vi "EminemGlobals.vi"() -> ()   [LabVIEW 2023]
uses:
  EminemStatesEnum.ctl
panel:
  out "ShooterSpeedRPM_FB":dbl=4000.0
  out "RShooterMotorOutput":dbl
  out "LShooterMotorOutput":dbl
  out "RShooterFilteredSpeed":dbl
  out "RShooterSpeed":dbl
  out "LShooterFilteredSpeed":dbl
  out "LShooterSpeed":dbl
  out "M&M_State":T1=enum."13-AmpDone"
  out "RAtSpeed":bool
  out "LAtSpeed":bool
  out "ShooterSensor":bool
  out "IntakeSensor":bool
  out "IntakeGetNoteMotorDMD":dbl=0.5
  out "ShooterSpeedRPM":dbl=4000.0
  out "ReadyForCommand":bool
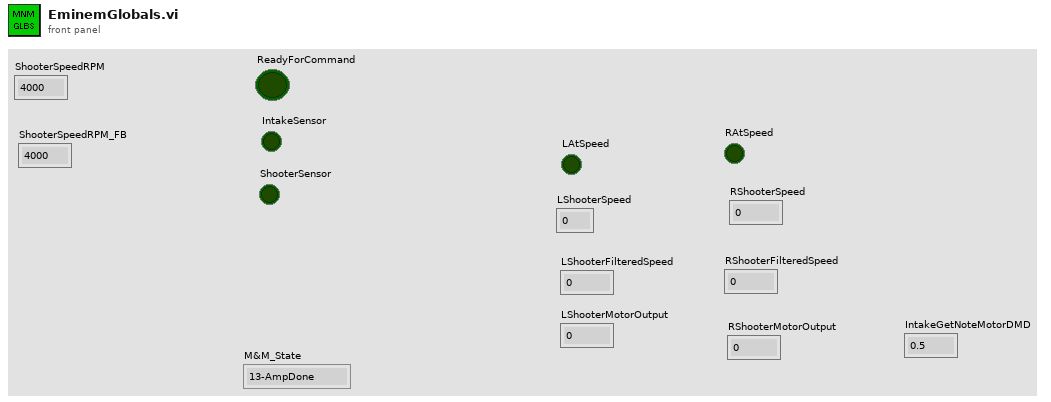
[diagram p1: front panel]
types:
  T1 = typedef "EminemStatesEnum.ctl" = enum16{"0-Init", "1-WaitForCmd", "2-Cancel", "3-ShootStart", "4-ShootRev", "5-ShootUpToSpd?", "6-ShootStartFeed&Timer", "7-ShootTimerOrSensorDone", "8-ShootDone", "9-AmpStart", "10-AmpUpToSpd?", "11-AmpStartFeed&Timer", "12-AmpTimerOrSensorDone", "13-AmpDone"}
diagram:
